vi "4155C Take SampleI v3.0.vi"(6 "Sample I - Drain/Gate":u32(ring)=1 items=["SMU1  ", "SMU2  ", "SMU3  ", "SMU4  ", "SMU5  ", "SMU6  ", "VSU1  ", "VSU2  "], 7 "Emergency Stop":refnum<vi>, 8 "error in (no error)":errorcluster, 9 "Idg 2":dbl min=-100.0 max=100.0 format="%.15e", 10 "Vdg compliance 2":dbl min=-100.0 max=100.0 format="%.15e", 11 "VISA resource name in":refnum<visa-resource-name>) -> (0 "error out":errorcluster, 1 "Idg":dbl[](array[numeric]) format="%.2f", 2 "Vdg":dbl[](array[numeric]) format="%.2f", 3 "VISA Resource Name out":refnum<visa-resource-name>, 4 "Is":dbl[](array[numeric]) format="%.2f", 5 "Time":dbl[](array[numeric]) format="%.2f")   [LabVIEW 2019]
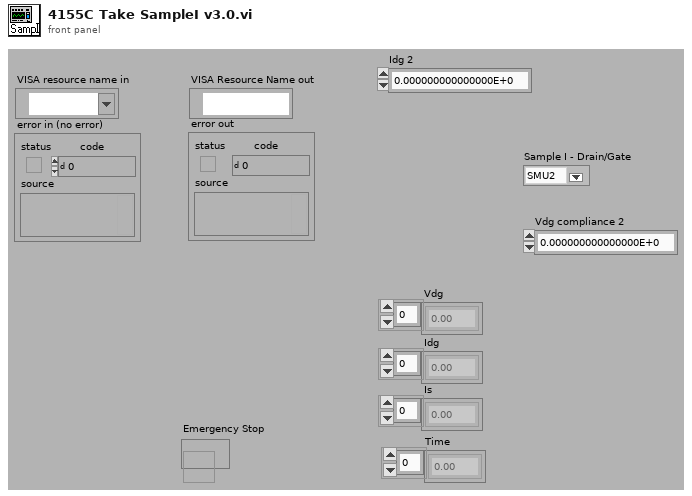
[diagram p1: front panel]
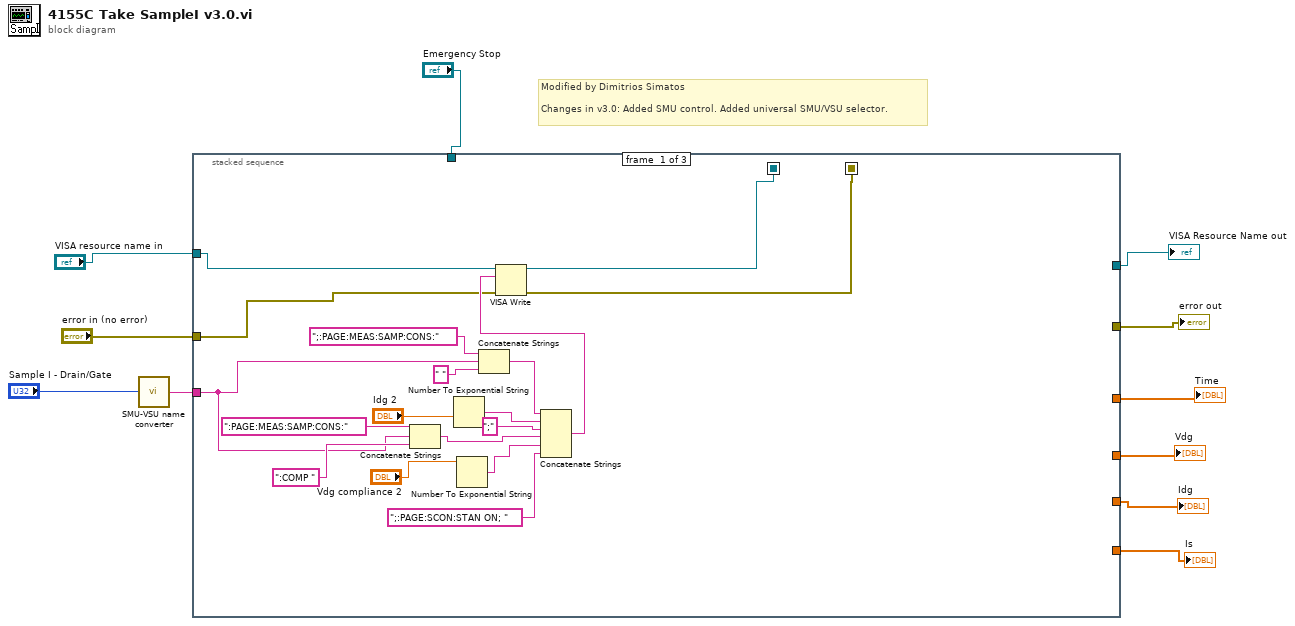
[diagram p0: block diagram]
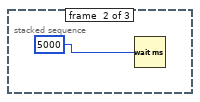
[diagram p2: hidden frame]
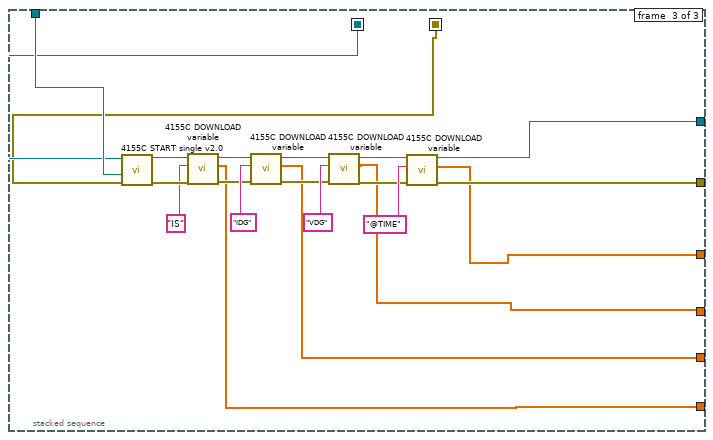
[diagram p3: hidden frame]
diagram:
  # "Modified by Dimitrios Simatos\n\nChanges in v3.0: Added SMU control. Added universal SMU/VSU selector."
  n1 = call "SMU-VSU name converter.vi"("unit to configure"="Sample I - Drain/Gate") -> ("SMU/VSU to be configured"=w1:string)
  n2 = stacked-sequence {
    seq-local: [w20 _ _] -> [_ _ w32]
    seq-local: [w19 _ _] -> [_ _ w31]
    tunnel: "Emergency Stop" -> [_ _ w39]
    tunnel: "VISA resource name in" -> [w23 _ _]
    tunnel: "error in (no error)" -> [w22 _ _]
    tunnel: [_ _ w38] -> w8
    tunnel: [_ _ w37] -> w7
    tunnel: [_ _ w36] -> w6
    tunnel: [_ _ w35] -> w5
    tunnel: [_ _ w34] -> w4
    tunnel: [_ _ w33] -> w3
    tunnel: w1 -> [w13 _ _]
    frame #0 {
      n3 = Concatenate Strings(":PAGE:MEAS:SAMP:CONS:" ("write buffer (\"\")"), w13, ":COMP " ("write buffer (\"\")")) -> (w16:string)
      n4 = Number To Exponential String(number="Idg 2") -> (E-format string=w25:string)  [unwired: 3 in]
      n5 = Number To Exponential String(number="Vdg compliance 2") -> (E-format string=w28:string)  [unwired: 3 in]
      n6 = Concatenate Strings(";:PAGE:MEAS:SAMP:CONS:" ("write buffer (\"\")"), w13, " " ("string")) -> (w17:string)
      n7 = Concatenate Strings(w17, w25, ";" ("Substring"), w16, w28, ";:PAGE:SCON:STAN ON; " ("write buffer (\"\")")) -> (w26:string)
      n8 = VISA Write(VISA resource name=w23, write buffer=w26, error in (no error)=w22) -> (VISA resource name out=w20:refnum<visa-resource-name>, error out=w19:errorcluster)  [unwired: 1 out]
    }
    frame #1 {
      n9 = Wait (ms)(milliseconds to wait=5000) -> ()  [unwired: 1 out]
    }
    frame #2 {
      n10 = call "4155C START single v2.0.vi"("error in (no error)"=w31, "Emergency Stop"=w39, "VISA resource name in"=w32) -> ("error out"=w50:errorcluster, "VISA Resource Name out"=w51:refnum<visa-resource-name>)  [unwired: 3 in]
      n11 = call "4155C DOWNLOAD variable.vi"("error in (no error)"=w50, "Variable name"="IS", "VISA resource name in"=w51) -> ("error out"=w47:errorcluster, "Output data"=w33:dbl[], "VISA Resource Name out"=w46:refnum<visa-resource-name>)  [unwired: 2 in]
      n12 = call "4155C DOWNLOAD variable.vi"("error in (no error)"=w47, "Variable name"="IDG", "VISA resource name in"=w46) -> ("error out"=w44:errorcluster, "Output data"=w34:dbl[], "VISA Resource Name out"=w43:refnum<visa-resource-name>)  [unwired: 2 in]
      n13 = call "4155C DOWNLOAD variable.vi"("error in (no error)"=w44, "Variable name"="VDG", "VISA resource name in"=w43) -> ("error out"=w40:errorcluster, "Output data"=w35:dbl[], "VISA Resource Name out"=w41:refnum<visa-resource-name>)  [unwired: 2 in]
      n14 = call "4155C DOWNLOAD variable.vi"("error in (no error)"=w40, "Variable name"="@TIME", "VISA resource name in"=w41) -> ("error out"=w37:errorcluster, "Output data"=w36:dbl[], "VISA Resource Name out"=w38:refnum<visa-resource-name>)  [unwired: 2 in]
    }
  }
  "VISA Resource Name out" <- w8
  "error out" <- w7
  "Time" <- w6
  "Vdg" <- w5
  "Idg" <- w4
  "Is" <- w3
